vi "Com_SECS Equipment _SECS Packet Flatten.vi"(8 "error in":errorcluster, 11 "SECS Packet":T1) -> (0 "error out":errorcluster, 3 "Data":string)   [LabVIEW 2016]
uses:
  Data Def/Com_SECS Equipment _SECS Packet.ctl
  Data Def/Com_SECS Equipment _Message Type.ctl
  Data Def/Com_SECS Equipment _Protocol Type.ctl
  Data Def/Com_SECS Equipment _Stream Type.ctl
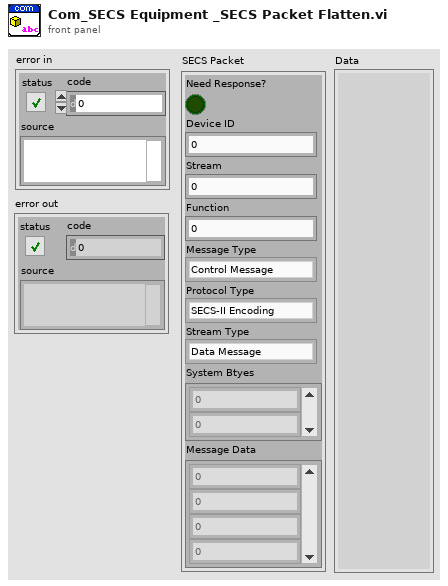
[diagram p1: front panel]
types:
  T1 = typedef "Com_SECS Equipment _SECS Packet.ctl" = cluster{"Need Response?":bool, "Device ID":u16, "Stream":u8, "Function":u8, "Message Type":T2, "Protocol Type":T3, "Stream Type":T4, "System Btyes":u8[], "Message Data":u8[]}
  T2 = typedef "Com_SECS Equipment _Message Type.ctl" = enum16{"Control Message", "Data Message"}
  T3 = typedef "Com_SECS Equipment _Protocol Type.ctl" = enum16{"SECS-II Encoding", "Reserved"}
  T4 = typedef "Com_SECS Equipment _Stream Type.ctl" = enum16{"Data Message", "Select.req", "Select.rsp", "Deselect.req", "Deselect.rsp", "Linktest.req", "Linktest.rsp", "Reject.req", "Separate.req", "Reserve"}
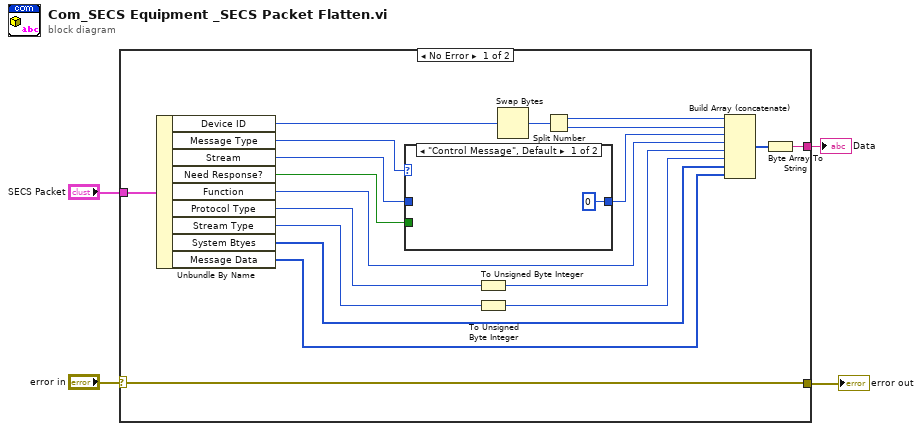
[diagram p0: block diagram]
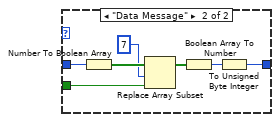
[diagram p2: hidden frame]
diagram:
  n1 = case shown="No Error" "error in" {
    selector: "error in" -> [w6 w32]
    tunnel: "SECS Packet" -> [w23 _]
    tunnel: [w6 w32] -> w2
    tunnel: [w5 _] -> w1
    frame No Error {
      n2 = Unbundle By Name(w23) -> ("Device ID"=w22:u16, "Message Type"=w18:T2, "Stream"=w17:u8, "Need Response?"=w16:bool, "Function"=w14:u8, "Protocol Type"=w13:T3, "Stream Type"=w11:T4, "System Btyes"=w9:u8[], "Message Data"=w8:u8[])
      n3 = case shown="\"Control Message\", Default" w18 {
        tunnel: w17 -> [_ w31]
        tunnel: w16 -> [_ w28]
        tunnel: [u8 0 w25] -> w15
        frame "Control Message", Default {
        }
        frame "Data Message" {
          n4 = Number To Boolean Array(number=w31) -> (Boolean array=w30:bool[])
          n5 = Replace Array Subset(array=w30, new element=w28, index=7) -> (w27:bool[])
          n6 = Boolean Array To Number(Boolean array=w27) -> (number=w26:u32)
          n7 = To Unsigned Byte Integer(number=w26) -> (unsigned 8bit integer=w25:u8)
        }
      }
      n8 = To Unsigned Byte Integer(number=w13) -> (unsigned 8bit integer=w12:u8)
      n9 = To Unsigned Byte Integer(number=w11) -> (unsigned 8bit integer=w10:u8)
      n10 = Swap Bytes(anything=w22) -> (byte swapped=w21:u16)
      n11 = Split Number(x=w21) -> (hi(x)=w20:u8, lo(x)=w19:u8)
      n12 = Build Array (concatenate)(w20, w19, w15, w14, w12, w10, w9, w8) -> (w7:u8[])
      n13 = Byte Array To String(unsigned byte array=w7) -> (string=w5:string)
    }
    frame Error {
    }
  }
  "error out" <- w2
  "Data" <- w1
